vi "Read String Configuration.vi"(8 "error in (no error)":errorcluster, 9 "Default If Not Found":string, 10 "Name":string, 11 "database-configuration in":refnum<class "configuration-database.lvclass">) -> (0 "error out":errorcluster, 1 "Not Found?":bool, 2 "Value":string, 3 "database-configuration out":refnum<class "configuration-database.lvclass">)   [LabVIEW 2020, in "configuration-database.lvlib" / "configuration-database.lvclass"]
uses:
  configuration-database.lvclass
  configuration-database.lvclass/configuration-database.ctl
  467ee455-6887-4cb9-9d84-75d0df8ab861.vi
  <vilib>/Utility/error.llb/Error Cluster From Error Code.vi
  IConfigDBQueries/IConfigurationDatabaseQueries.lvclass
  externals/database-interface/IDatabase/IDatabase/IDatabase.lvclass
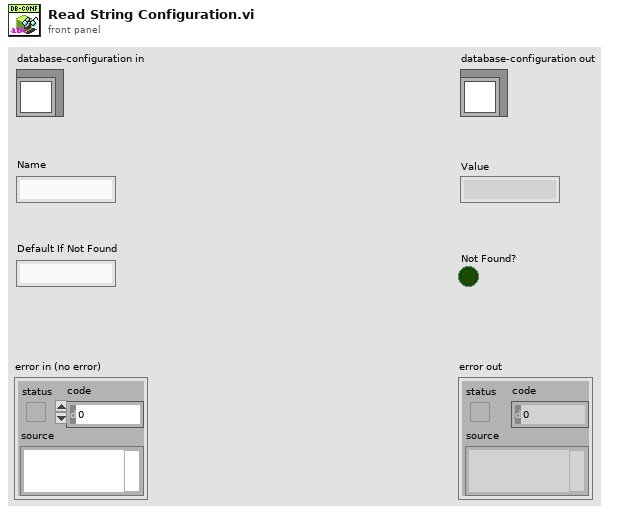
[diagram p1: front panel]
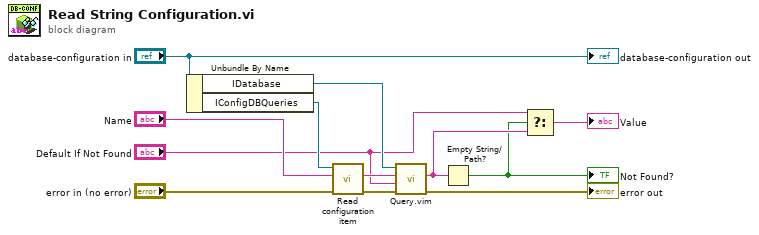
[diagram p0: block diagram]
diagram:
  n1 = Unbundle By Name("database-configuration in") -> ("IDatabase"=w11:refnum<class "IDatabase.lvclass">, "IConfigDBQueries"=w12:refnum<class "IConfigurationDatabaseQueries.lvclass">)
  n2 = call-dynamic "Read configuration item.vi"("error in (no error)"="error in (no error)", "configuration item"="Name", "IConfigDBQueries in"=w12) -> ("error out"=w10:errorcluster, "result"=w9:string)  [unwired: 7 in]
  n3 = call "Query.vim"("error in (no error)"=w10, "Type and Default"="Default If Not Found", "Query string"=w9, "IDatabase in"=w11) -> ("error out"=→"error out":errorcluster, "Result"=w7:string)  [unwired: 5 in, 1 out]
  n4 = Empty String/Path?(string/path=w7) -> (empty?=w3:bool)
  "Not Found?" <- w3
  n5 = Select(t="Default If Not Found", s=w3, f=w7) -> (s? t:f=→"Value":string)
  "database-configuration out" <- "database-configuration in"
